vi "pad with zeroes.vi"(2 "String 2 input":string, 3 "String 1 input":string) -> (0 "String 2 output":string, 1 "String 1 output":string)   [LabVIEW 2009]
doc: "This takes two strings (presumably of 0s and 1s), and pads the shorter one with zeroes so that it has the same length as the longer one."
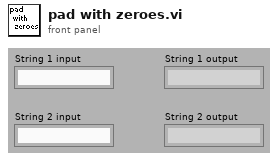
[diagram p1: front panel]
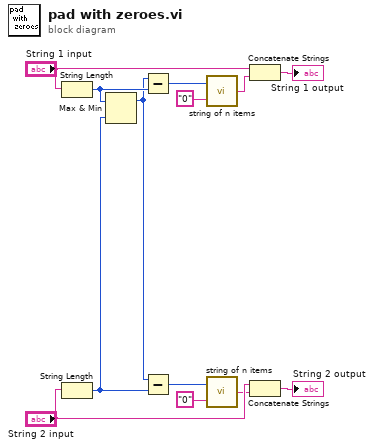
[diagram p0: block diagram]
diagram:
  n1 = String Length(string="String 1 input") -> (length=w2:i32)
  n2 = String Length(string="String 2 input") -> (length=w3:i32)
  n3 = Max & Min(x=w2, y=w3) -> (max(x,y)=w1:i32)  [unwired: 1 out]
  n4 = Subtract(x=w1, y=w2) -> (x-y=w5:i32)
  n5 = Subtract(x=w1, y=w3) -> (x-y=w7:i32)
  n6 = call "string of n items.vi"("string"="0", "Numeric"=w5) -> ("String"=w8:string)
  n7 = call "string of n items.vi"("string"="0", "Numeric"=w7) -> ("String"=w9:string)
  n8 = Concatenate Strings("String 1 input", w8) -> (→"String 1 output":string)
  n9 = Concatenate Strings("String 2 input", w9) -> (→"String 2 output":string)
